vi "AddSingleSingle.vi"(7 "Priority":refnum<class "Action.lvclass">, 10 "Standard":refnum<class "Action.lvclass">, 11 "ActionStack in":refnum<class "Action.lvclass">[](array[class])) -> (3 "ActionStack out":refnum<class "Action.lvclass">[](array[class]))   [LabVIEW 2024, in "ActionStack.lvlib" / "Action.lvclass"]
uses:
  Action.lvclass
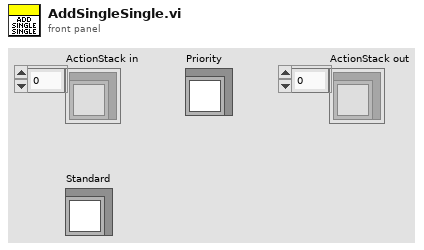
[diagram p1: front panel]
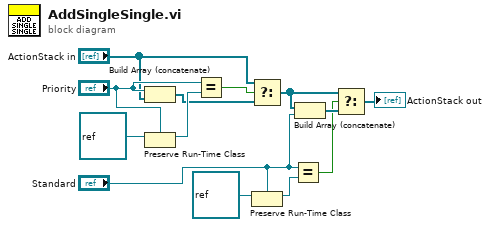
[diagram p0: block diagram]
diagram:
  n1 = Build Array (concatenate)("Priority", "ActionStack in") -> (w6:refnum<class "Action.lvclass">[])
  n2 = Preserve Run-Time Class(object in=refnum<class> refnum, 2:"Priority") -> (object out=w10:refnum<class "Action.lvclass">)  [unwired: 1 in, 1 out]
  n3 = Equal?(x="Priority", y=w10) -> (x = y?=w8:bool)
  n4 = Select(t="ActionStack in", s=w8, f=w6) -> (s? t:f=w3:refnum<class "Action.lvclass">[])
  n5 = Preserve Run-Time Class(object in=refnum<class> refnum, 2:"Standard") -> (object out=w12:refnum<class "Action.lvclass">)  [unwired: 1 in, 1 out]
  n6 = Equal?(x="Standard", y=w12) -> (x = y?=w2:bool)
  n7 = Build Array (concatenate)(w3, "Standard") -> (w4:refnum<class "Action.lvclass">[])
  n8 = Select(t=w3, s=w2, f=w4) -> (s? t:f=→"ActionStack out":refnum<class "Action.lvclass">[])
